vi "readFromXML.vi"(8 "error in (no error)":errorcluster, 10 "XML in":string="<AOSPointingOffset>\n\t\t<xCorrection_arcsec>111</xCorrection_arcsec>\n\t\t<yCorrection_arcsec>12</yCorrection_arcsec>\n</AOSPointingOffset>\n", 11 "ADCWavelength in":refnum<class "ADCWavelength.lvclass">) -> (0 "error out":errorcluster, 3 "ADCWavelength out":refnum<class "ADCWavelength.lvclass">)   [LabVIEW 2014, in "TCSDataDefinitions.lvlib" / "TCSAtmosphericDispersionCommand.lvlib" / "ADCWavelength.lvclass"]
uses:
  ADCWavelength.lvclass
  <userlib>/Common/UnitsAndXML/FlattenItemWithUnitToXML/FlattenLengthToXML/LengthUnit.ctl
  ADCWavelength.lvclass/ADCWavelength.ctl
  TCSAtmosphericDispersionCommand/TCSAtmosphericDispersionCommand.lvclass
  <userlib>/Common/UnitsAndXML/UnitsAndXML.lvlib
  <userlib>/Common/XML/XMLParser/XMLParser.lvclass
panel:
  out "wavelength1":dbl[unit]
  out "wavelength2":dbl[unit]
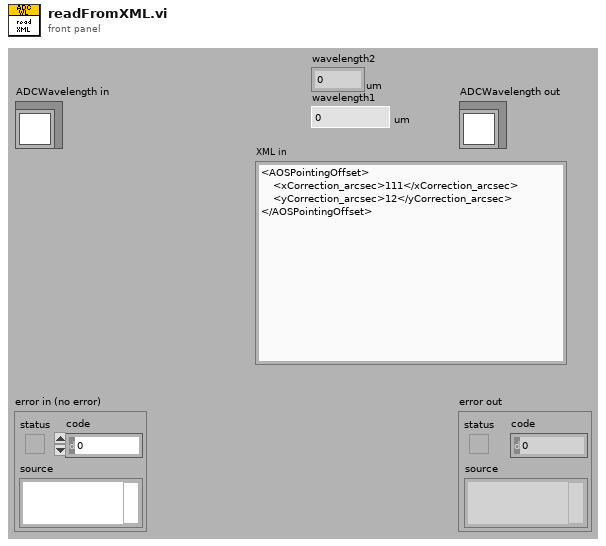
[diagram p1: front panel]
types:
  T1 = typedef "UnitsAndXML.lvlib/LengthUnit.ctl" = enum16{"m", "Angstrom", "AU", "chain", "cm", "cubit", "fathom", "fermi", "ft", "furlong", "hubble", "in", "ly", "mi", "mm", "rod", "um", "yd"}
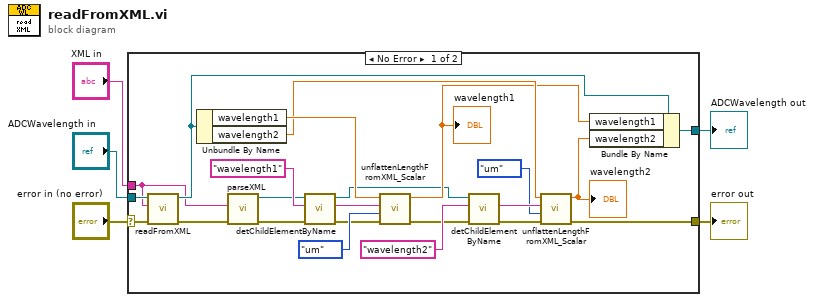
[diagram p0: block diagram]
diagram:
  n1 = case shown="No Error" "error in (no error)" {
    selector: "error in (no error)" -> [w17 w30]
    tunnel: [w16 w30] -> w4
    tunnel: [w14 w29] -> w2
    tunnel: "ADCWavelength in" -> [w28 w29]
    tunnel: "XML in" -> [w12 _]
    frame No Error {
      n2 = call-parent "readFromXML.vi"("error in (no error)"=w17, "XML in"=w12, "TCSAtmosphericDispersionCommand in"=w28) -> ("error out"=w26:errorcluster, "TCSAtmosphericDispersionCommand out"=w15:refnum<class "ADCWavelength.lvclass">)  [unwired: 7 in]
      n3 = Unbundle By Name(w15) -> ("wavelength1"=w21:dbl[unit], "wavelength2"=w20:dbl[unit])
      n4 = call <userlib>:"parseXML.vi"("error in (no error)"=w26, "XMLString in"=w12) -> ("error out"=w27:errorcluster, "Element out"=w10:refnum<class "XMLParser.lvclass">)  [unwired: 8 in]
      n5 = call <userlib>:"detChildElementByName.vi"("error in (no error)"=w27, "childName"="wavelength1" ("ChildName"), "Element in"=w10) -> ("error out"=w7:errorcluster, "childXML"=w23:string, "Element out"=w9:refnum<class "XMLParser.lvclass">)  [unwired: 5 in, 1 out]
      n6 = call <userlib>:"unflattenLengthFromXML_Scalar.vi"("error in (no error)"=w7, "lengthUnitInXML"=LengthUnit."um", "xmlString"=w23, "lengthForType"=w21) -> ("error out"=w6:errorcluster, "length"=w13:dbl[unit])  [unwired: 6 in]
      "wavelength1" <- w13
      n7 = call <userlib>:"detChildElementByName.vi"("error in (no error)"=w6, "childName"="wavelength2" ("ChildName"), "Element in"=w9) -> ("error out"=w8:errorcluster, "childXML"=w22:string)  [unwired: 5 in, 2 out]
      n8 = call <userlib>:"unflattenLengthFromXML_Scalar.vi"("error in (no error)"=w8, "lengthUnitInXML"=LengthUnit."um", "xmlString"=w22, "lengthForType"=w20) -> ("error out"=w16:errorcluster, "length"=w11:dbl[unit])  [unwired: 6 in]
      "wavelength2" <- w11
      n9 = Bundle By Name(cluster=w15, "wavelength1"=w13, "wavelength2"=w11) -> (w14:refnum<class "ADCWavelength.lvclass">)
    }
    frame Error {
    }
  }
  "error out" <- w4
  "ADCWavelength out" <- w2
